vi "Keyence.Cmd.TuneQuit.vi"(8 "error in (no error)":errorcluster, 9 "Timeout [ms] (1000)":i32=1000, 11 "cID in":refnum<k5>) -> (0 "error out":errorcluster, 1 "cmd ok":bool, 2 "tune quitted":bool, 3 "cID out":refnum<k5>)   [LabVIEW 2016]
panel:
  out "response":string
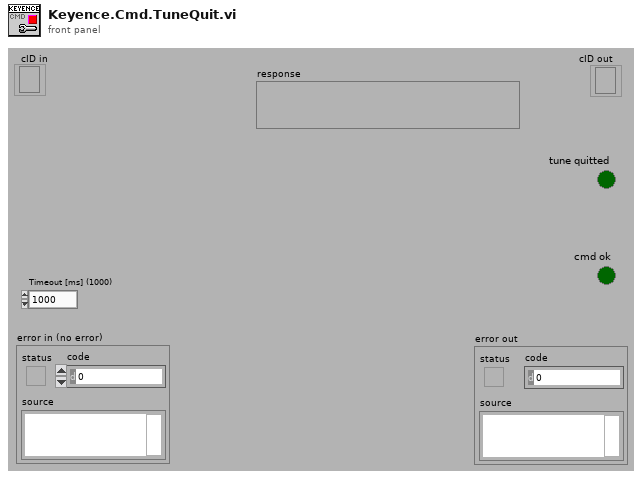
[diagram p1: front panel]
types:
  T1 = enum16{"Standard", "Buffered", "CRLF", "Immediate"}
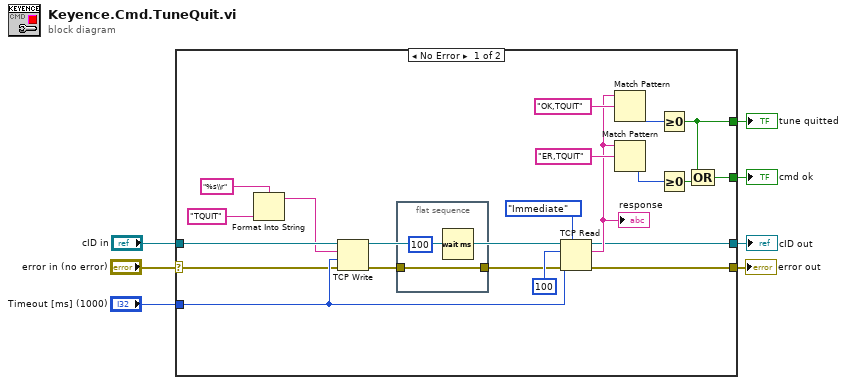
[diagram p0: block diagram]
diagram:
  n1 = case shown="No Error" "error in (no error)" {
    selector: "error in (no error)" -> [w12 w32]
    tunnel: [w22 w32] -> w7
    tunnel: "Timeout [ms] (1000)" -> [w28 _]
    tunnel: [w16 _] -> w4
    tunnel: [w14 _] -> w3
    tunnel: "cID in" -> [w13 w31]
    tunnel: [w8 w31] -> w1
    frame No Error {
      n2 = Format Into String(format string="%s\\r" ("data in"), "TQUIT" ("data in")) -> (resulting string=w9:string)  [unwired: 2 in, 1 out]
      n3 = TCP Write(connection ID=w13, data in=w9, error in (no error)=w12, 9:w28) -> (connection ID out=w27:refnum<k5>, error out=w24:errorcluster)  [unwired: 1 out]
      n4 = flat-sequence {
        tunnel: w24 -> [w30]
        tunnel: [w30] -> w23
        frame #0 {
          n5 = Wait (ms)(milliseconds to wait=u32 100) -> ()  [unwired: 1 out]
        }
      }
      n6 = TCP Read(connection ID=w27, bytes to read=100, error in (no error)=w23, 7:T1."Immediate" ("mode (standard)"), 9:w28) -> (connection ID out=w8:refnum<k5>, data out=w15:string, error out=w22:errorcluster)
      "response" <- w15
      n7 = Match Pattern(string=w15, regular expression="OK,TQUIT") -> (offset past match=w17:i32)  [unwired: 1 in, 3 out]
      n8 = Match Pattern(string=w15, regular expression="ER,TQUIT") -> (offset past match=w20:i32)  [unwired: 1 in, 3 out]
      n9 = Greater Or Equal To 0?(x=w17) -> (x >= 0?=w14:bool)
      n10 = Greater Or Equal To 0?(x=w20) -> (x >= 0?=w19:bool)
      n11 = Compound Arithmetic op=OR(w14, w19) -> (w16:bool)
    }
    frame Error {
    }
  }
  "error out" <- w7
  "cmd ok" <- w4
  "tune quitted" <- w3
  "cID out" <- w1
